vi "Temp FGV.vi"(0 "TableIn":string[][](array[string])=[["Default", "", "", " 0"], ["Case1", "", "", "1"], ["Case2", "", "", "2"], ["Case3", "", "", "3"], ["Case4", "", "", "4"], ["Case5", "", "", "5"], ["Case6", "", "", "6"], ["Case7", "", "", "7"], ["Case8", "", "", "8"], ["Case9", "", "", "9"], ["Case10", "", "", "10"], ["", "", "", ""], ["", "", "", ""], ["", "", "", ""], ["", "", "", ""], ["", "", "", ""], ["", "", "", ""], ["", "", "", ""], ["", "", "", ""], ["", "", "", ""], ["", "", "", ""], ["22", "", "", ""], ["23", "", "", ""], ["24", "", "", ""], ["25", "", "", ""]], 1 "Action":T1(ring)=enum."WrteAll", 5 "X":i32, 7 "Y":i32, 9 "DataIn":string, 11 "error in":errorcluster) -> (4 "TableOut":string[][](array[string]), 10 "DataOut":string, 15 "error out":errorcluster)   [LabVIEW 2019]
uses:
  09bdc40f-24f8-42fa-be14-94a5734f4f81.vi
  3a88f7dc-0fdf-4cec-95e5-a4f3429e1c34.vi
  Commonly VI/Main Glb.vi
  <vilib>/JDP Science/JSONtext/Variant to JSON Text.vi
  <vilib>/JDP Science/JSONtext/JSON text to Variant.vi
  Commonly VI.lvlib
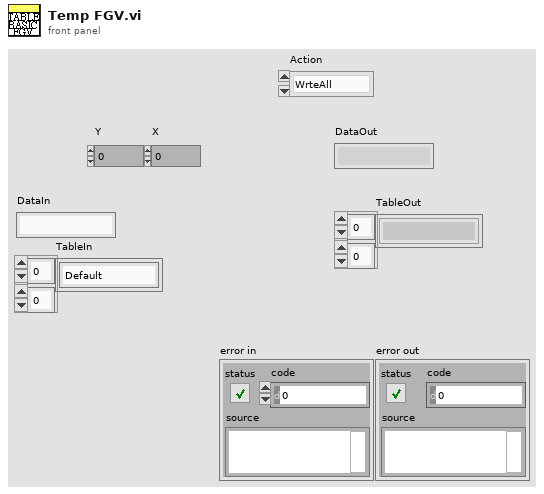
[diagram p1: front panel]
types:
  T1 = enum16{"Initial", "Write", "Read", "Save", "Load", "WrteAll"}
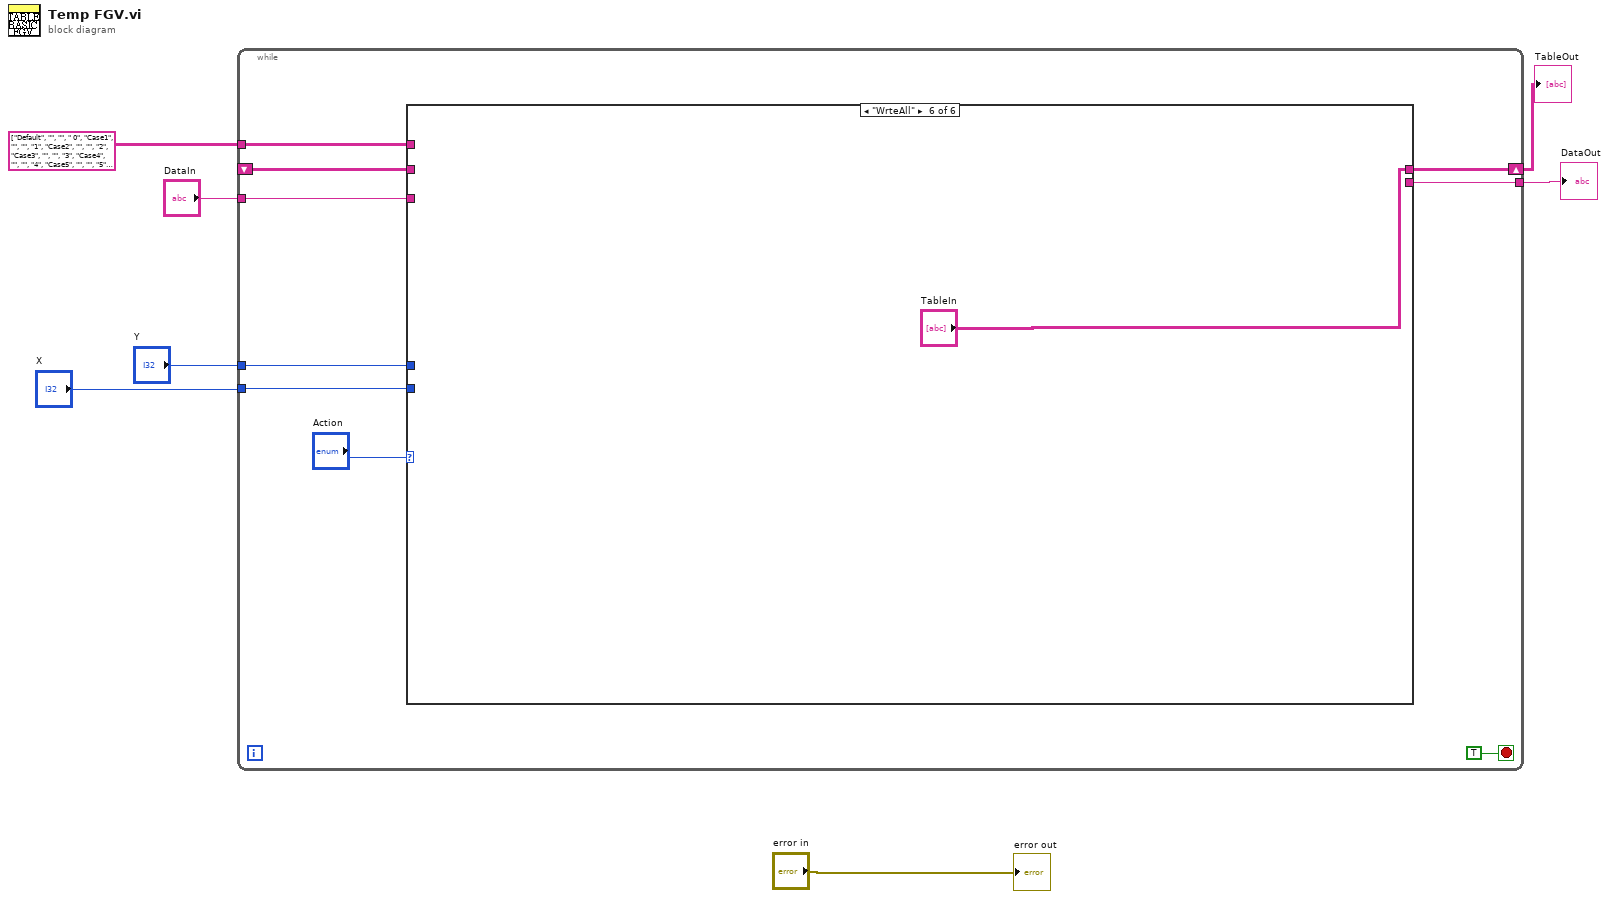
[diagram p0: block diagram]
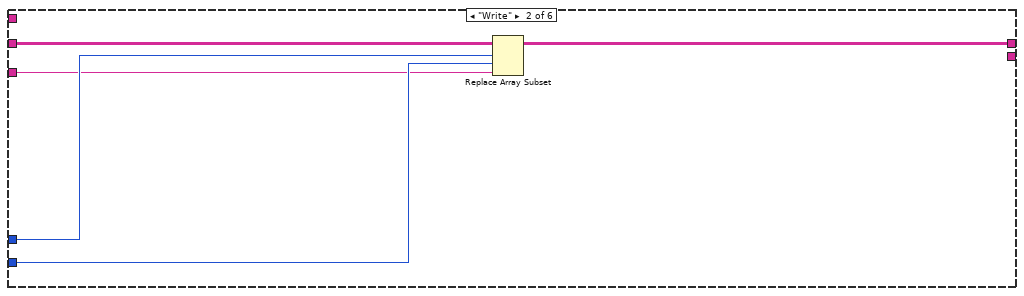
[diagram p3: hidden frame]
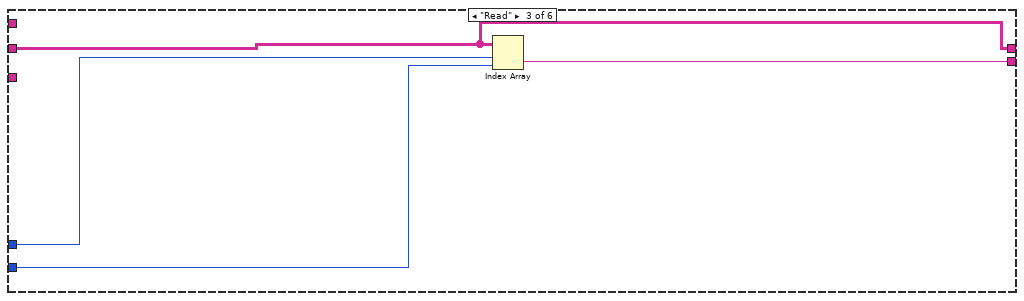
[diagram p4: hidden frame]
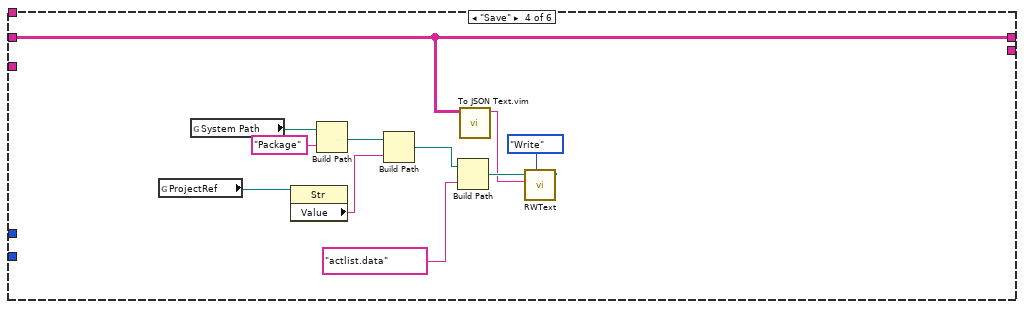
[diagram p5: hidden frame]
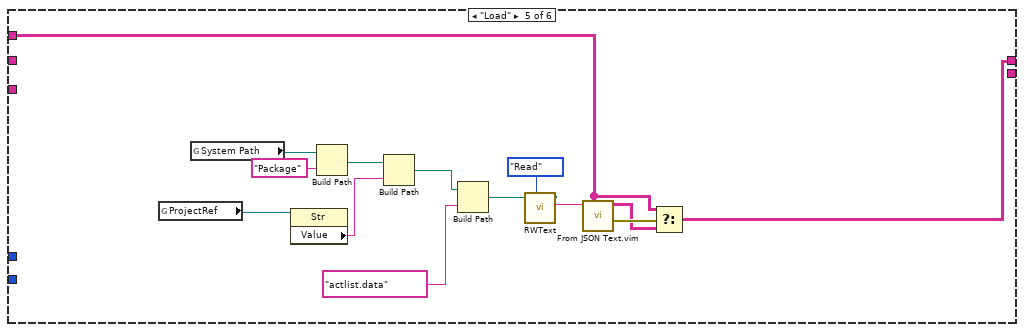
[diagram p6: hidden frame]
diagram:
  n1 = while {
    shift-right: [w16] -> w2
    shift-left: _ -> [w15]
    tunnel: string[][] [["Default", "", "", " 0"], ["Case1", "", "", "1"], ["Case2", "", "", "2"], ["Case3", "", "", "3"], ["Case4", "", "", "4"], ["Case5", "", "", "5"], ["Case6", "", "", "6"], ["Case7", "", "", "7"], ["Case8", "", "", "8"], ["Case9", "", "", "9"], ["Case10", "", "", "10"], ["", "", "", ""], ["", "", "", ""], ["", "", "", ""], ["", "", "", ""], ["", "", "", ""], ["", "", "", ""], ["", "", "", ""], ["", "", "", ""], ["", "", "", ""], ["", "", "", ""], ["22", "", "", ""], ["23", "", "", ""], ["24", "", "", ""], ["25", "", "", ""]] ("Item Names") -> [w14]
    tunnel: "X" -> [w12]
    tunnel: "Y" -> [w11]
    tunnel: "DataIn" -> [w10]
    tunnel: [w8] -> w6
    stop <- TRUE stop-if-true
    n2 = case shown="\"WrteAll\"" "Action" {
      tunnel: [w17 w22 w24 w28 w38 "TableIn"] -> w16
      tunnel: w15 -> [_ w21 w24 w28 _ _]
      tunnel: w14 -> [w17 _ _ _ w40 _]
      tunnel: w12 -> [_ w20 w26 _ _ _]
      tunnel: w11 -> [_ w19 w25 _ _ _]
      tunnel: w10 -> [_ w18 _ _ _ _]
      tunnel: [_ _ w23 _ _ _] -> w8
      frame "Initial", Default {
      }
      frame "Write" {
        n3 = Replace Array Subset(array=w21, new element=w18, index (row)=w19, index (col)=w20) -> (w22:string[][])
      }
      frame "Read" {
        n4 = Index Array(array=w24, index (row)=w25, index (col)=w26) -> (element=w23:string)
      }
      frame "Save" {
        n5 = global read "Main Glb.vi" "ProjectRef"() -> (w34:refnum<vi>)
        n6 = global read "Main Glb.vi" "System Path"() -> (w37:path)
        n7 = property class="Str"(reference=w34) -> ("Value"=w33:string)  [unwired: 1 in, 2 out]
        n8 = Build Path(base path=w37, name or relative path="Package") -> (appended path=w35:path)
        n9 = Build Path(base path=w35, name or relative path=w33) -> (appended path=w31:path)
        n10 = Build Path(base path=w31, name or relative path="actlist.data") -> (appended path=w29:path)
        n11 = call "To JSON Text.vim"("Anything"=w28) -> ("<JSON>"=w27:string)  [unwired: 9 in, 1 out]
        n12 = call "RWText.vi"("Action"=enum16{"Read", "Write"}."Write", "TextIn"=w27, "file path (use dialog)"=w29) -> ()  [unwired: 7 in, 2 out]
      }
      frame "Load" {
        n13 = global read "Main Glb.vi" "ProjectRef"() -> (w48:refnum<vi>)
        n14 = global read "Main Glb.vi" "System Path"() -> (w51:path)
        n15 = property class="Str"(reference=w48) -> ("Value"=w47:string)  [unwired: 1 in, 2 out]
        n16 = Build Path(base path=w51, name or relative path="Package") -> (appended path=w49:path)
        n17 = Build Path(base path=w49, name or relative path=w47) -> (appended path=w45:path)
        n18 = Build Path(base path=w45, name or relative path="actlist.data") -> (appended path=w43:path)
        n19 = call "RWText.vi"("Action"=enum16{"Read", "Write"}."Read", "file path (use dialog)"=w43) -> ("textOut"=w42:string)  [unwired: 8 in, 1 out]
        n20 = call "From JSON Text.vim"("Data Type and Default Value"=w40, "JSON"=w42) -> ("error out"=w41:errorcluster, "Data out"=w39:string[][])  [unwired: 8 in]
        n21 = Select(t=w40, s=w41, f=w39) -> (s? t:f=w38:string[][])
      }
      frame "WrteAll" {
      }
    }
  }
  "DataOut" <- w6
  "TableOut" <- w2
  "error out" <- "error in"
